vi "Attach Error Source.vi"(6 "Delete Call Chain?":bool, 8 "Error In":errorcluster, 10 "Error Source":T1=enum."< --- Modules --- >") -> (0 "Error Out":errorcluster, 1 "Call Chain":string, 2 "Source":string)   [LabVIEW 2019, in "Error.lvclass"]
uses:
  Error.lvclass
  SubModules/LogsAbstract/TypeDef/Event Source.ctl
  a458d2e6-0cdc-46bd-8e17-6b252ab13941.vi
  <vilib>/Utility/Data Type/Get Numeric Information.vi
  SubModules/LogsAbstract/LogsAbstract.lvclass
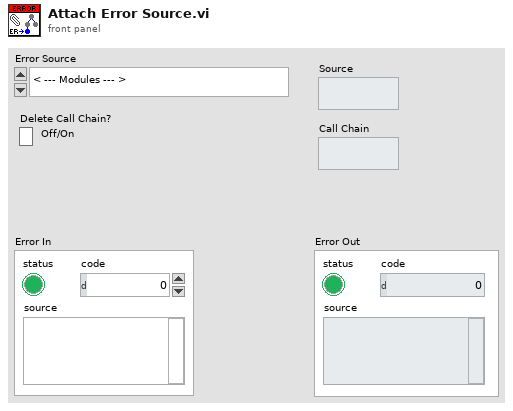
[diagram p1: front panel]
types:
  T1 = typedef "LogsAbstract.lvlib/LogsAbstract.lvclass/Event Source.ctl" = enum16{"Unknown", "< --- Modules --- >", "Core", "< --- SubModules --- >", "EventLog -> Core", "ErrorLog -> Core"}
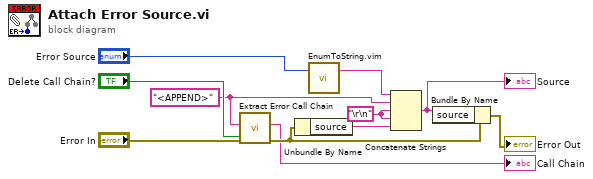
[diagram p0: block diagram]
diagram:
  w1 = "<APPEND>" ("string")
  w8 = "\r\n"
  n1 = call "Extract Error Call Chain.vi"("Delete Call Chain?"="Delete Call Chain?", "Error In"="Error In", "Search Tag"=w1) -> ("Error Out"=w4:errorcluster, "Read Call Chain"=→"Call Chain":string)  [unwired: 7 in]
  n2 = Unbundle By Name(w4) -> ("source"=w6:string)
  n3 = call "EnumToString.vim"("Enum"="Error Source") -> ("Enum Value"=w10:string)  [unwired: 16 in, 2 out]
  n4 = Concatenate Strings(w10, w1, w8, w8, w6) -> (w7:string)
  "Source" <- w7
  n5 = Bundle By Name(cluster=w4, "source"=w7) -> (→"Error Out":errorcluster)
